vi "Setup.SingleNodeBrowser.Init.vi"(8 "error in (no error)":errorcluster, 11 "Variables":T1 {"NIVS.DisplayFilter" items=["K_CHAN_R", "K_CHAN_W", "K_CHAN_RW", "K_CHAN_VOLT", "K_CHAN_FAULT", "K_ALL", "K_CUSTOM", "K_CHAN_R_VIS", "K_CHAN_W_VIS", "K_CHAN_RW_VIS", "K_CHAN_VOLT_VIS", "K_CHAN_FAULT_VIS"]}) -> (0 "error out":errorcluster, 3 "Cluster out":T1 {"NIVS.DisplayFilter" items=["K_CHAN_R", "K_CHAN_W", "K_CHAN_RW", "K_CHAN_VOLT", "K_CHAN_FAULT", "K_ALL", "K_CUSTOM", "K_CHAN_R_VIS", "K_CHAN_W_VIS", "K_CHAN_RW_VIS", "K_CHAN_VOLT_VIS", "K_CHAN_FAULT_VIS"]})   [LabVIEW 2015, in "Workspace.Obejct.Radio.lvlib"]
uses:
  Workspace.Obejct.Radio.lvlib
  Types/Setup.StateVariables.ctl
  <vilib>/NI Veristand/UI Controls/Single Node Browser/Net Event Data.ctl
  <vilib>/NI Veristand/UI Controls/Single Node Browser/Net Event.ctl
  Types/Config.ctl
  NationalInstruments.VeriStand.SystemStorage
  NationalInstruments.VeriStand.SystemStorageUI
  <vilib>/Utility/miscctls.llb/LVRowAndColumnTypeDef.ctl
  <vilib>/NI Veristand/UI Controls/Single Node Browser/NI_VS UI Single Node Browser.lvlib
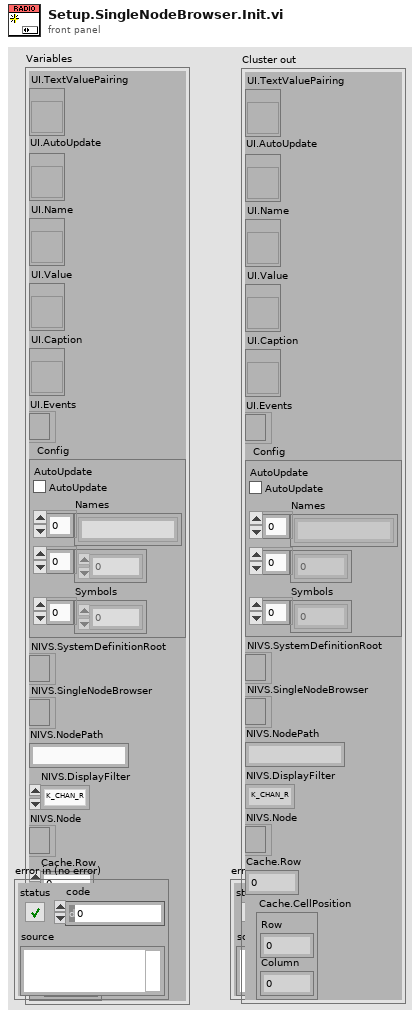
[diagram p1: front panel]
types:
  T1 = typedef "Workspace.Obejct.Radio.lvlib/Setup.StateVariables.ctl" = cluster{"UI.TextValuePairing":refnum<vi>, "UI.AutoUpdate":refnum<vi>, "UI.Name":refnum<vi>, "UI.Value":refnum<vi>, "UI.Caption":refnum<vi>, "UI.Events":refnum<event-registration>, "Config":T2, "NIVS.SystemDefinitionRoot":refnum<k24>, "NIVS.SingleNodeBrowser":refnum<k24>, "NIVS.NodePath":string, "NIVS.DisplayFilter":u8, "NIVS.Node":refnum<k24>, "Cache.Row":i32, "Cache.CellPosition":T3}
  T2 = typedef "Workspace.Obejct.Radio.lvlib/Config.ctl" = cluster{"AutoUpdate":bool, "Names":string[], "Values":dbl[], "Symbols":i32[]}
  T3 = typedef "LVRowAndColumnTypeDef.ctl" = cluster{"Row":i32, "Column":i32}
  T4 = typedef "NI_VS UI Single Node Browser.lvlib/Callback Type.ctl" = cluster{"Net Callbacks":refnum<k27>[], "Event":refnum<user-event>}
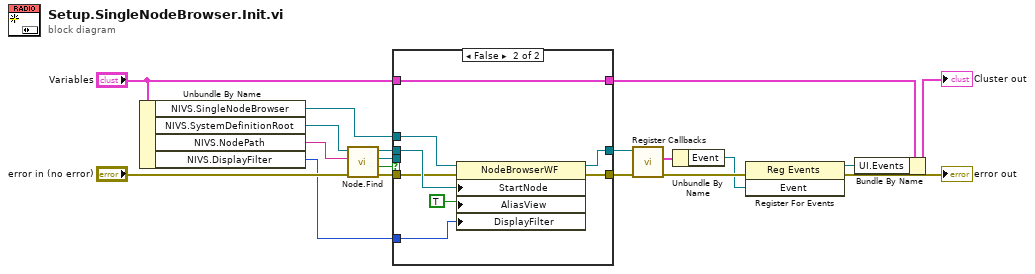
[diagram p0: block diagram]
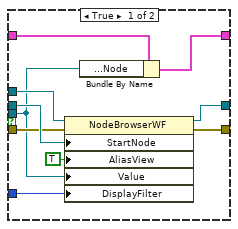
[diagram p2: hidden frame]
diagram:
  n1 = Unbundle By Name("Variables") -> ("NIVS.SingleNodeBrowser"=w15:refnum<k24>, "NIVS.SystemDefinitionRoot"=w14:refnum<k24>, "NIVS.NodePath"=w13:string, "NIVS.DisplayFilter"=w12:u8)
  n2 = call "Node.Find.vi"("error in (no error)"="error in (no error)", "nodePath"=w13, "System Def Root"=w14) -> ("error out"=w3:errorcluster, "FindNode"=w9:bool, "Node"=w10:refnum<k24>, "System Def Root"=w11:refnum<k24>)  [unwired: 5 in]
  n3 = case shown="False" w9 {
    tunnel: w12 -> [w26 w31]
    tunnel: w15 -> [w29 w37]
    tunnel: [w23 w36] -> w7
    tunnel: w11 -> [w28 w35]
    tunnel: w3 -> [w27 w34]
    tunnel: w10 -> [w21 _]
    tunnel: [w24 w33] -> w8
    tunnel: "Variables" -> [w22 w30]
    tunnel: [w20 w30] -> w1
    frame True {
      n4 = property class="NodeBrowserWF"(reference=w29, error in=w27, "StartNode"=w28, "AliasView"=TRUE, "Value"=w21, "DisplayFilter"=w26) -> (reference out=w24:refnum<k24>, error out=w23:errorcluster)
      n5 = Bundle By Name(cluster=w22, "NIVS.Node"=w21) -> (w20:T1)
    }
    frame False {
      n6 = property class="NodeBrowserWF"(reference=w37, error in=w34, "StartNode"=w35, "AliasView"=TRUE, "DisplayFilter"=w31) -> (reference out=w33:refnum<k24>, error out=w36:errorcluster)
    }
  }
  n7 = call <vilib>:"Register Callbacks.vi"("error in (no error)"=w7, "Single Node Browser"=w8) -> ("error out"=w6:errorcluster, "Callbacks"=w4:T4)  [unwired: 7 in, 1 out]
  n8 = Unbundle By Name(w4) -> ("Event"=w5:refnum<user-event>)
  n9 = register-events(error in=w6, w5) -> (reference out=w17:refnum<event-registration>, error out=→"error out":errorcluster)  [unwired: 1 in]
  n10 = Bundle By Name(cluster=w1, "UI.Events"=w17) -> (→"Cluster out":T1)
